vi "Write Global Locked.vi"(8 "error in (no error)":errorcluster, 10 "Global":refnum<class "System.lvclass">, 11 "System in":refnum<class "System.lvclass">) -> (0 "error out":errorcluster, 3 "System out":refnum<class "System.lvclass">)   [LabVIEW 2013, in "System.lvclass"]
uses:
  System.lvclass
  System.lvclass/System.ctl
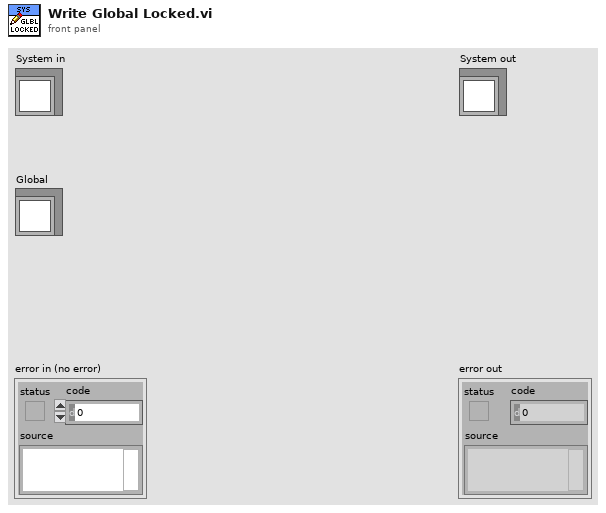
[diagram p1: front panel]
types:
  T1 = typedef "Semaphore RefNum" = refnum<k1>
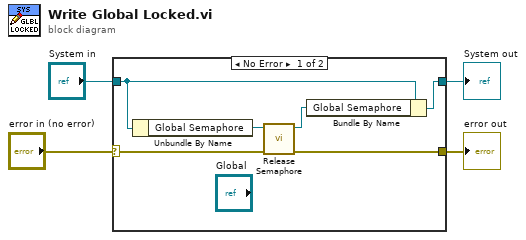
[diagram p0: block diagram]
diagram:
  n1 = case shown="No Error" "error in (no error)" {
    selector: "error in (no error)" -> [w6 w12]
    tunnel: [w5 w12] -> w3
    tunnel: [w8 w11] -> w1
    tunnel: "System in" -> [w10 w11]
    frame No Error {
      n2 = Unbundle By Name(w10) -> ("Global Semaphore"=w9:T1)
      n3 = call <vilib>:"Release Semaphore.vi"("error in (no error)"=w6, "semaphore"=w9) -> ("error out"=w5:errorcluster, "semaphore out"=w7:T1)  [unwired: 4 in]
      n4 = Bundle By Name(cluster=w10, "Global Semaphore"=w7) -> (w8:refnum<class "System.lvclass">)
    }
    frame Error {
    }
  }
  "error out" <- w3
  "System out" <- w1
